vi "VariantToSGL.vi"(11 "Element":variant) -> (3 "Numeric":sgl)   [LabVIEW 2016, in "DSI-RT.lvlib"]
uses:
  DSI-RT.lvlib
  <vilib>/Utility/Data Type/NI_Data Type.lvlib
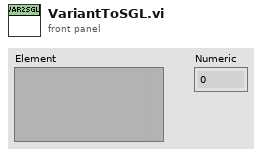
[diagram p1: front panel]
types:
  T1 = typedef "NI_Data Type.lvlib/Data Type.ctl" = enum8{"Invalid Type", "Void", "I8", "I16", "I32", "I64", "U8", "U16", "U32", "U64", "Single Float", "Double Float", "Extended Float", "Single Complex", "Double Complex", "Extended Complex", "Enum U8", "Enum U16", "Enum U32", "Enum U64", "Single Float With Unit", "Double Float With Unit", "Extended Float With Unit", "Single Complex with Unit", "Double Complex with Unit", "Extended Complex with Unit", "Boolean", "String", "Path", "Picture", "Tag", "Array", "Cluster", "Variant", "LV Variant", "Waveform", "Timestamp", "Digital Waveform", "Digital Data", "ExpressData", "Refnum", "External Data", "VI", "Poly VI", "LabVIEW Class Instance", "Fixed Point"}
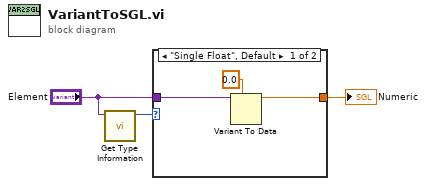
[diagram p0: block diagram]
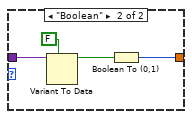
[diagram p2: hidden frame]
diagram:
  n1 = call <vilib>:"Get Type Information.vi"("Variant"="Element") -> ("Type"=w1:T1)  [unwired: 6 in, 4 out]
  n2 = case shown="\"Single Float\", Default" w1 {
    tunnel: [w6 w7] -> w3
    tunnel: "Element" -> [w4 w8]
    frame "Single Float", Default {
      n3 = Variant To Data(type=sgl 0.0, Variant=w4) -> (data=w6:sgl)  [unwired: 1 in, 1 out]
    }
    frame "Boolean" {
      n4 = Variant To Data(type=FALSE, Variant=w8) -> (data=w10:bool)  [unwired: 1 in, 1 out]
      n5 = Boolean To (0,1)(Boolean=w10) -> (0, 1=w7:i16)
    }
  }
  "Numeric" <- w3
